vi "SystemLink_Test_Eric.vi"() -> ()   [LabVIEW 2020]
uses:
  Summer2020/LabVIEWCode/Subs/Server XCtrl/Server.xctl
  Summer2020/LabVIEWCode/Subs/ColorText/Code.xctl
  Summer2020/LabVIEWCode/Subs/SystemLink/SL_Subs/SL_XControl.xctl
  Summer2020/LabVIEWCode/Subs/SystemLink/SL_Subs/SystemLink_Write_String.vi
panel:
  out "REPL":string="\n...         try:\n...             s = s + fred.readline()\n...         except:\n...             utime.sleep(0.1)\n...     # print(s)\n... \nTraceback (most recent call last):\n  File \"<stdin>\", line 5\nSyntaxError: invalid syntax\n>>> \n>>> comm(request)\nTraceback (most recent call last):\n  File \"<stdin>\", line 1, in <module>\nNameError: name 'comm' isn't defined\n>>> \n>>> s =  b''\n>>> fred.write(b_string + eol)\nurequest(\"apple.com\")web24\n"
  out "value of Bill":string="Yo Bill"
  in  "String":string="Yo Bill"
  in  "SL_XControl 2":string(xcontrol)="Bill"
  in  "SL_XControl":string(xcontrol)
  in  "Code":string(xcontrol)="import hub,utime\nfred = hub.USB_VCP()\n\nrequest = b'urequest(\"apple.com\")'\neol = b'web'\nreol = b'back'\n\ndef comm(b_string):\n    s =  b''\n    fred.write(b_string + eol)\n    while not(reol in s):\n        try:\n            s = s + fred.readline()\n        except:\n            utime.sleep(0.1)\n    # print(s)\n\ncomm(request)\n\ns =  b''\nfred.write(b_string + eol)\n    while not(reol in s):\n        try:\n            s = s + fred.readline()\n        except:\n            utime.sleep(0.1)\n       print(s)\n    "
  in  "Server":path(xcontrol)=path "E:/Chris/_2020 Spring/Summer2020/Summer2020/LabVIEWCode/Servers/Jens.vi"
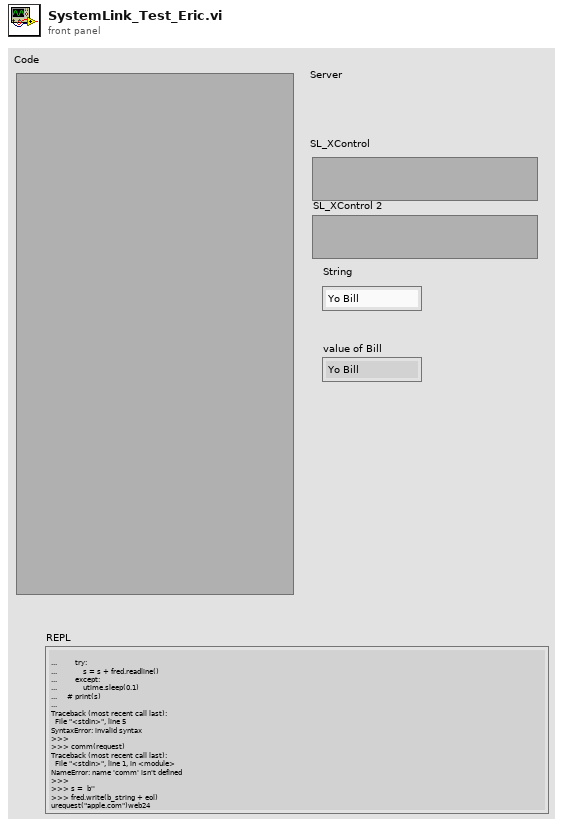
[diagram p1: front panel]
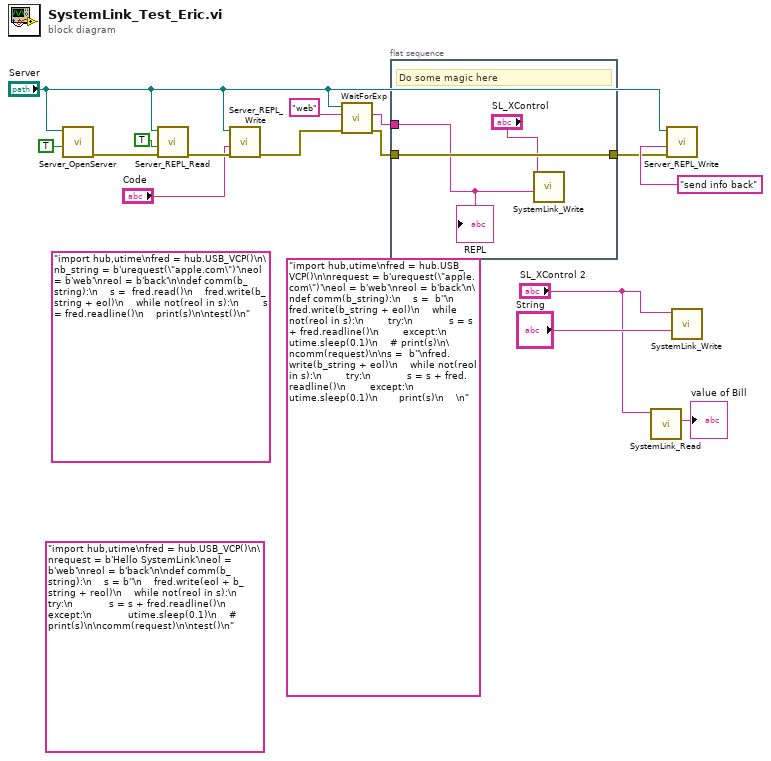
[diagram p0: block diagram]
diagram:
  (unwired) "import hub,utime\nfred = hub.USB_VCP()\n\nrequest = b'Hello SystemLink'\neol = b'web'\nreol = b'back'\n\ndef comm(b_string):\n    s = b''\n    fred.write(eol + b_string + reol)\n    while not(reol in s):\n        try:\n            s = s + fred.readline()\n        except:\n            utime.sleep(0.1)\n    # print(s)\n\ncomm(request)\n\ntest()\n" ("Code")
  (unwired) "import hub,utime\nfred = hub.USB_VCP()\n\nrequest = b'urequest(\"apple.com\")'\neol = b'web'\nreol = b'back'\n\ndef comm(b_string):\n    s =  b''\n    fred.write(b_string + eol)\n    while not(reol in s):\n        try:\n            s = s + fred.readline()\n        except:\n            utime.sleep(0.1)\n    # print(s)\n\ncomm(request)\n\ns =  b''\nfred.write(b_string + eol)\n    while not(reol in s):\n        try:\n            s = s + fred.readline()\n        except:\n            utime.sleep(0.1)\n       print(s)\n    \n" ("Code")
  (unwired) "import hub,utime\nfred = hub.USB_VCP()\n\nb_string = b'urequest(\"apple.com\")'\neol = b'web'\nreol = b'back'\n\ndef comm(b_string):\n    s =  fred.read()\n    fred.write(b_string + eol)\n    while not(reol in s):\n        s = fred.readline()\n    print(s)\n\ntest()\n" ("Code")
  n1 = call "Server_OpenServer.vi"("Wait for connection?"=TRUE, "Server"="Server") -> ("error out"=w13:errorcluster)  [unwired: 9 in]
  n2 = call "Server_REPL_Read.vi"("error in (no error)"=w13, "Clear"=TRUE, "Server"="Server") -> ("error out"=w12:errorcluster)  [unwired: 6 in, 2 out]
  n3 = call "Server_REPL_Write.vi"("error in (no error)"=w12, "Code"="Code", "Server"="Server") -> ("error out"=w15:errorcluster)  [unwired: 8 in]
  n4 = call "WaitForExp.vi"("error in (no error)"=w15, "expression"="web" ("regular expression"), "Server"="Server") -> ("error out"=w6:errorcluster, "REPL"=w3:string)  [unwired: 7 in]
  n5 = flat-sequence {
    tunnel: [w18] -> w7
    tunnel: w6 -> [w18]
    tunnel: w3 -> [w17]
    frame #0 {
      # "Do some magic here"
      n6 = call-poly "SystemLink_Write.vi"("String"=w17, "SL_XControl"="SL_XControl") -> ()  [unwired: 9 in, 1 out]
      "REPL" <- w17
    }
  }
  n7 = call "SystemLink_Read.vi"("SystemLink Tag"="SL_XControl 2") -> ("value"=→"value of Bill":string)  [unwired: 7 in, 3 out]
  n8 = call "Server_REPL_Write.vi"("error in (no error)"=w7, "Code"="send info back" ("Command"), "Server"="Server") -> ()  [unwired: 8 in, 1 out]
  n9 = call-poly "SystemLink_Write.vi"("String"="String", "SL_XControl"="SL_XControl 2") -> ()  [unwired: 9 in, 1 out]
